vi "SetValue.vi"(8 "error in (no error)":errorcluster, 10 "Value":dbl, 11 "DAQmx-AI":refnum<class "DAQmx-AI.lvclass">) -> (0 "error out":errorcluster, 3 "DAQmx-AI out":refnum<class "DAQmx-AI.lvclass">)   [LabVIEW 2016, in "DAQmx-AI.lvclass"]
doc: "---------------------------------------------------------------\nJKI State Machine Objects™\nhttp://jki.net/state-machine-objects/\nCopyright (C) 2005-2015, JKI <info@jki.net>\nALL RIGHTS RESERVEDJKI State Machine Objects (SMO) 1.0.0.5\nJKI - JKI\nCopyright (c) 2016, JKI"
uses:
  DAQmx-AI.lvclass
  DAQmx-AI.lvclass/DAQmx-AI.ctl
  Typedefs/DataChanged--EventData--Cluster.ctl
panel:
  # "For instructions on how to use the JKI State Machine Objects, examples and video tutorials, visit:\nhttp://jki.net/state-machine-objects/\n\nJKI State Machine Objects™\nhttp://jki.net/state-machine-objects/\nCopyright (C) 2005-2015, JKI <info@jki.net>\nALL RIGHTS RESERVED"
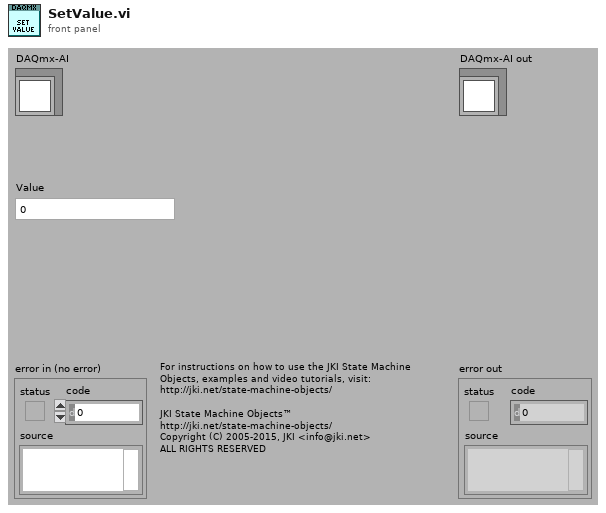
[diagram p1: front panel]
types:
  T1 = typedef "DAQmx-AI.lvclass/DataChanged--EventData--Cluster.ctl" = cluster{"Timestamp":timestamp, "Value":dbl}
  T2 = typedef "DAQmx-AI.lvclass/PrivateData--Ref.ctl" = refnum<data-value>
  T3 = typedef "DAQmx-AI.lvclass/PrivateData--Cluster.ctl" = cluster{"Configuration":T4, "Public Events":T6, "Data":dbl, "Scaling":T7, "Private Events":T13}
  T4 = typedef "DAQmx-AI.lvclass/Configuration--Cluster.ctl" = cluster{"PhysChan":tag, "Period (ms)":i64, "input terminal cfg":i32, "minimum value":dbl, "maximum value":dbl, "units":T5, "task name":string, "TDMS File Path":path, "Group Name":string}
  T5 = typedef "DAQmx-AI.lvclass/Units -- Enum.ctl" = enum16{"Volts", "Amps", "Deg F", "Deg C", "Deg R", "Kelvins", "Strain", "Ohms", "Hz", "Seconds", "Meters", "Inches", "Degrees", "Radians", "Ticks", "g", "m/s^2", "m/s", "in/s", "Pascals", "Newtons", "Pounds", "kgf", "psi", "bar", "Nm", "oz-in", "lb-in", "lb-ft", "Volts/Volt", "mVolts/Volt", "From TEDS"}
  T6 = typedef "DAQmx-AI.lvclass/PublicEvents--Cluster.ctl" = cluster{"Value Changed":refnum<user-event>, "Task Configuration":refnum<user-event>, "Scaling":refnum<user-event>}
  T7 = typedef "DAQmx-AI.lvclass/Scaling--Cluster.ctl" = cluster{"Scale Name":string, "Scale Type":T8, "Scaled Units":string, "Linear":T9, "Map Range":T10, "Polynomial":T11, "Table":T12}
  T8 = typedef "DAQmx-AI.lvclass/ScalingType--Enum.ctl" = enum16{"No scaling", "Linear", "Map Range", "Polynomial", "Table"}
  T9 = typedef "DAQmx-AI.lvclass/Scaling(Linear)--Cluster.ctl" = cluster{"Slope":dbl, "Intercept":dbl}
  T10 = typedef "DAQmx-AI.lvclass/Scaling(MapRange)--Cluster.ctl" = cluster{"Minimum":dbl, "Maximum":dbl}
  T11 = typedef "DAQmx-AI.lvclass/Scaling(Polynomial)--Cluster.ctl" = cluster{"forward coeff":dbl[], "reverse coeff":dbl[]}
  T12 = typedef "DAQmx-AI.lvclass/Scaling(Table)--Cluster.ctl" = cluster{"scaled values":dbl[], "pres-scaled values":dbl[]}
  T13 = typedef "DAQmx-AI.lvclass/PrivateEvents--Cluster.ctl" = cluster{"Logging":refnum<user-event>}
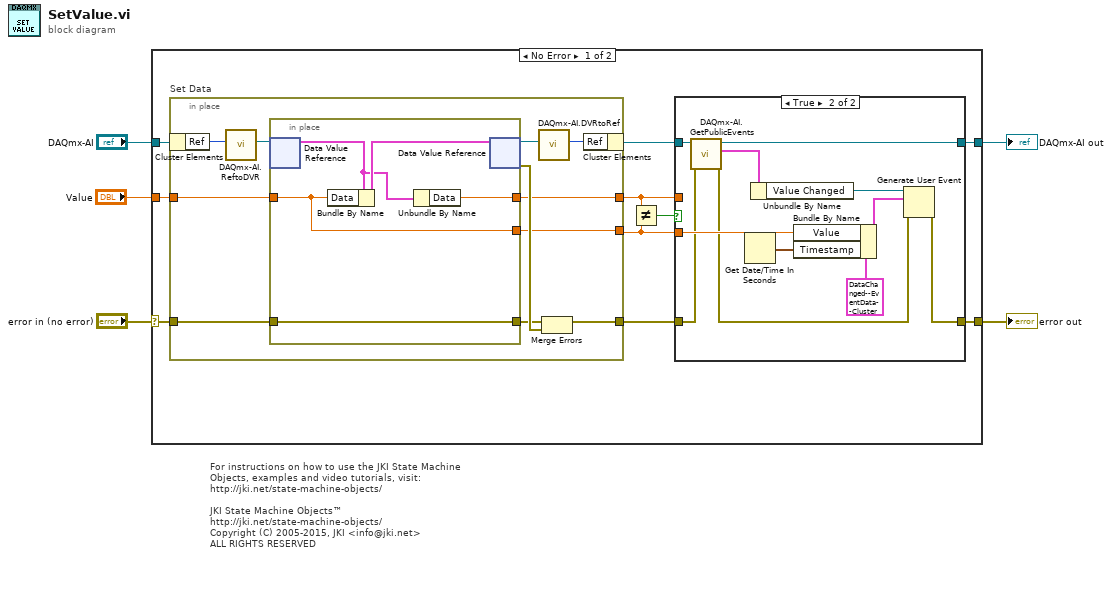
[diagram p0: block diagram]
diagram:
  # "For instructions on how to use the JKI State Machine Objects, examples and video tutorials, visit:\nhttp://jki.net/state-machine-objects/\n\nJKI State Machine Objects™\nhttp://jki.net/state-machine-objects/\nCopyright (C) 2005-2015, JKI <info@jki.net>\nALL RIGHTS RESERVED"
  n1 = case shown="No Error" "error in (no error)" {
    selector: "error in (no error)" -> [w13 w45]
    tunnel: "DAQmx-AI" -> [w14 w46]
    tunnel: [w11 w45] -> w4
    tunnel: [w6 w46] -> w3
    tunnel: "Value" -> [w15 _]
    frame No Error {
      n2 = in-place "Set Data" {
        in-place-border: w13 -> [w39]
        in-place-border: [w36] -> w12
        in-place-border: w15 -> [w35]
        in-place-border: [w34] -> w8
        in-place-border: [w33] -> w9
        n3 = in-place-cluster #1(w14) -> ("Ref"=w32:u32)
        n4 = call "DAQmx-AI.ReftoDVR.vi"("Ref"=w32) -> ("Ref"=w31:T2)  [unwired: 10 in]
        n5 = in-place {
          in-place-border: w39 -> [w44]
          in-place-border: [w44] -> w37
          in-place-border: w35 -> [w42]
          in-place-border: [w42] -> w34
          in-place-border: [w41] -> w33
          n6 = in-place-dvr #2(w31) -> (w40:T3)  [unwired: 1 out]
          n7 = Bundle By Name(cluster=w40, "Data"=w42) -> (w43:T3)
          n8 = Unbundle By Name(w40) -> ("Data"=w41:dbl)
          n9 = in-place-dvr #2(w43) -> (w30:T2, w38:errorcluster)
        }
        n10 = call "DAQmx-AI.DVRtoRef.vi"("Ref"=w30) -> ("Ref"=w29:u32)  [unwired: 10 in]
        n11 = Merge Errors(w37, w38) -> (w36:errorcluster)
        n12 = in-place-cluster #1("Ref"=w29) -> (w10:refnum<class "DAQmx-AI.lvclass">)
      }
      n13 = Not Equal?(x=w9, y=w8) -> (x != y?=w7:bool)
      n14 = case shown="True" w7 {
        tunnel: w12 -> [w16 w21]
        tunnel: w9 -> [_ _]
        tunnel: w8 -> [_ w25]
        tunnel: [w16 w23] -> w11
        tunnel: w10 -> [w17 w22]
        tunnel: [w17 w19] -> w6
        frame False {
        }
        frame True {
          n15 = call "DAQmx-AI.GetPublicEvents.vi"("error in (no error)"=w21, "DAQmx-AI"=w22) -> ("error out"=w20:errorcluster, "DAQmx(AI) Public Events"=w18:T6, "DAQmx-AI out"=w19:refnum<class "DAQmx-AI.lvclass">)  [unwired: 7 in]
          n16 = Get Date/Time In Seconds() -> (seconds since 1Jan1904=w24:timestamp)
          n17 = Unbundle By Name(w18) -> ("Value Changed"=w28:refnum<user-event>)
          n18 = Bundle By Name(cluster=T1 {"Timestamp"=timestamp(0 s since 1904-01-01), "Value"=0.0} ("event data"), "Value"=w25, "Timestamp"=w24) -> (w26:T1)
          n19 = Generate User Event(user event=w28, event data cluster=w26, error in=w20) -> (error out=w23:errorcluster)  [unwired: 1 in, 1 out]
        }
      }
    }
    frame Error {
    }
  }
  "error out" <- w4
  "DAQmx-AI out" <- w3
